vi "setItemToolTip.vi"(8 "Error In":errorcluster, 9 "toolTip":string, 10 "index":i32, 11 "QToolBox In":refnum<class "QToolBox.lvclass">) -> (0 "Error Out":errorcluster, 3 "QToolBox Out":refnum<class "QToolBox.lvclass">)   [LabVIEW 2014, in "QToolBox.lvclass"]
doc: "LabVIEW-specific documentation is not yet available. See <b>http://doc.qt.io/qt-5/QToolBox.html#setItemToolTip</b>"
uses:
  QToolBox.lvclass
  LQ Core/LQIdentity/LQIdentity.lvclass/LQIdentity.ctl
  LQ Core/LQ Core.lvlib
  LQ Core/LQIdentity/LQIdentity.lvclass
panel:
  # "Copyright (c) 2016 Sze Howe Koh\n\nThis Source Code Form is subject to the terms of the Mozilla Public\nLicense, v. 2.0. If a copy of the MPL was not distributed with this\nfile, You can obtain one at http://mozilla.org/MPL/2.0/."
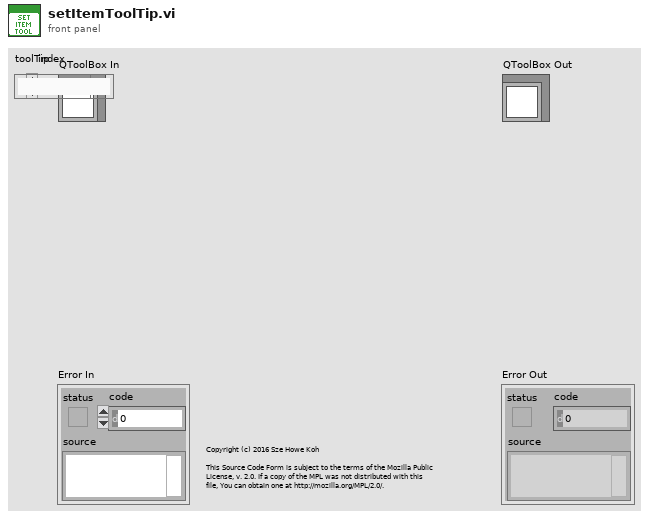
[diagram p1: front panel]
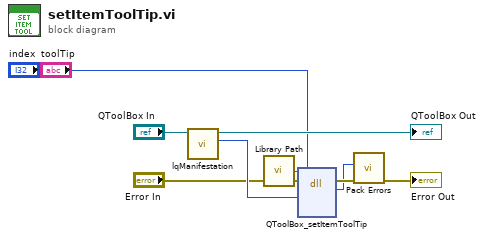
[diagram p0: block diagram]
diagram:
  n1 = call "lqManifestation.vi"("LQIdentity in"="QToolBox In") -> ("Manifestation"=w7:u64, "LQIdentity out"=→"QToolBox Out":refnum<class "QToolBox.lvclass">)  [unwired: 9 in]
  n2 = call "Library Path.vi"() -> ("Library Path"=w8:path)
  n3 = dll-call lib="?" fn="QToolBox_setItemToolTip"(path in=w8, error in="Error In", "_instance"=w7, "index"="index", "toolTip"="toolTip") -> (error out=w5:errorcluster, w3:i32)  [unwired: 4 in, 1 out]
  n4 = call "Pack Errors.vi"("Error In"=w5, "Error Code"=w3) -> ("Error Out"=→"Error Out":errorcluster)  [unwired: 9 in]
